vi "NML GPIB Tester.vi"(5 "String to write":string, 7 "Read":bool, 8 "Write":bool, 9 "VISA resource name":refnum<visa-resource-name>) -> (4 "String Read":string)   [LabVIEW 2024]
doc: "General LabView-GPIB VI which allows the selection of a message termination mode, timeout and usefule english error codes and status messages.\nScott Hannahs, FBNML, Feb 1993"
uses:
  <vilib>/Instr/_visa.llb/VISA GPIB Control REN Mode.ctl
panel:
  out "∆ Time (mS)":u32
  in  "Read Mode":u32(slide) scale=0.0..2.0
  in  "Write Mode":u32(slide) scale=0.0..5.0
  out "Error Out":errorcluster {"code" format="%.0x"}
  out "Write Status":string
  out "Read Status":string
  in  "Timeout (sec)":ext=1.0 format="%.1f"
  in  "Byte count":u32=2000
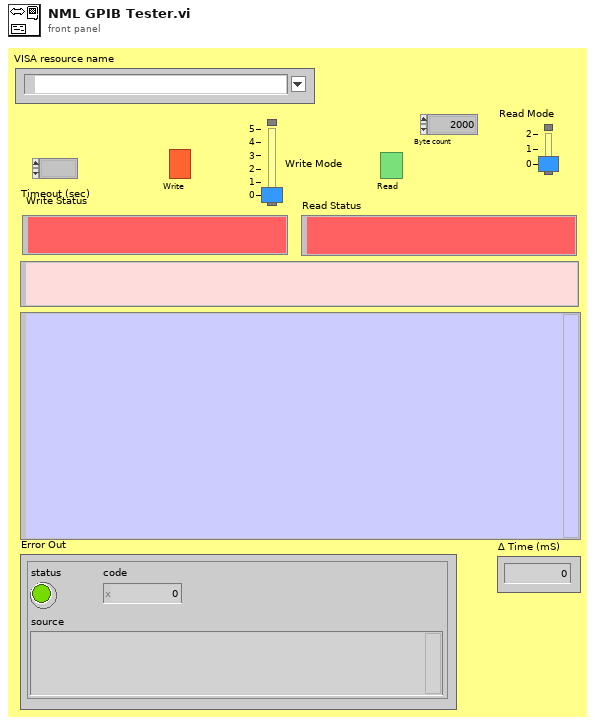
[diagram p1: front panel]
types:
  T1 = typedef "VISA GPIB Control REN Mode.ctl" = u16
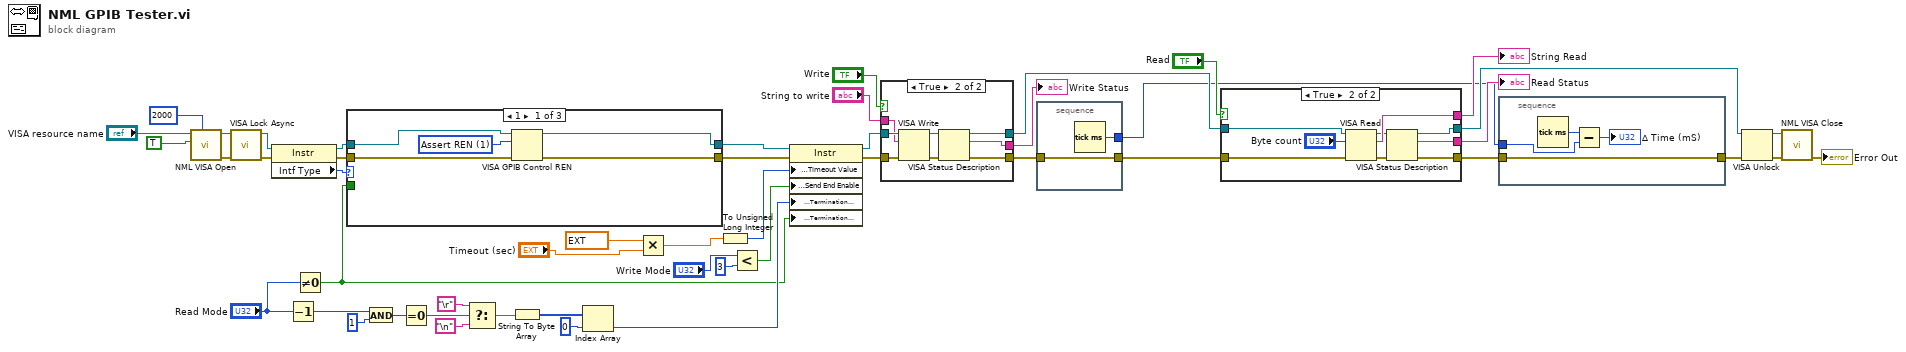
[diagram p0: block diagram]
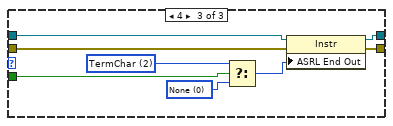
[diagram p3: hidden frame]
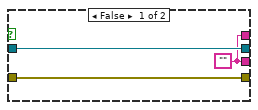
[diagram p4: hidden frame]
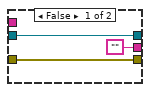
[diagram p5: hidden frame]
diagram:
  n1 = call "NML VISA Open.vi"("VISA Open timeout (0)"=u32 2000 ("timeout (0)"), "duplicate session (T)"=TRUE ("duplicate session (F)"), "VISA resource name"="VISA resource name") -> ("error out"=w8:errorcluster, "VISA resource name out"=w13:refnum<visa-resource-name>)  [unwired: 7 in]
  n2 = call <vilib>:"VISA Lock Async.vi"("error in (no error)"=w8, "VISA resource name"=w13) -> ("error out"=w7:errorcluster, "VISA resource name out"=w9:refnum<visa-resource-name>)  [unwired: 7 in, 1 out]
  n3 = property class="Instr"(reference=w9, error in=w7) -> (reference out=w11:refnum<visa-resource-name>, error out=w12:errorcluster, "Intf Type"=w2:u16)
  n4 = Decrement(x="Read Mode") -> (x-1=w29:u32)
  n5 = Not Equal To 0?(x="Read Mode") -> (x != 0?=w4:bool)
  n6 = case shown="1" w2 {
    tunnel: [w54 w56 w62] -> w15
    tunnel: [w53 w55 w61] -> w14
    tunnel: w12 -> [w52 w55 w63]
    tunnel: w11 -> [w51 w56 w64]
    tunnel: w4 -> [_ _ w58]
    frame 1 {
      w50 = T1 1 items=["Deassert REN", "Assert REN", "Go To Local; Deassert REN ", "Assert REN; Address Device", "Local Lockout (Addressed Devices)", "Local Lockout (This Device)", "Go To Local"] ("Mode")
      n7 = VISA GPIB Control REN(8:w52, 10:w50, 11:w51) -> (0:w53:errorcluster, 3:w54:refnum<visa-resource-name>)
    }
    frame Default {
    }
    frame 4 {
      w57 = u16 2 items=["None", "Last Bit", "TermChar", "Break"] ("Serial Settings:End Mode for Writes")
      w59 = u16 0 items=["None", "Last Bit", "TermChar", "Break"] ("Serial Settings:End Mode for Writes")
      n8 = Select(t=w57, s=w58, f=w59) -> (s? t:f=w60:u16)
      n9 = property class="Instr"(reference=w64, error in=w63, "ASRL End Out"=w60) -> (reference out=w62:refnum<visa-resource-name>, error out=w61:errorcluster)
    }
  }
  n10 = And(x=w29, y=u32 1) -> (x .and. y?=w31:u32)
  n11 = Equal To 0?(x=w31) -> (x = 0?=w32:bool)
  n12 = Select(t="\r", s=w32, f="\n") -> (s? t:f=w27:string)
  n13 = String To Byte Array(string=w27) -> (unsigned byte array=w26:u8[])
  n14 = Index Array(array=w26, index=0 ("Index")) -> (element=w22:u8)
  n15 = Multiply(x=ext 1000.0, y="Timeout (sec)") -> (x*y=w47:ext)
  n16 = To Unsigned Long Integer(number=w47) -> (unsigned 32bit integer=w41:u32)
  n17 = Less?(x="Write Mode", y=u32 3) -> (x < y?=w36:bool)
  n18 = property class="Instr"(reference=w15, error in=w14, "General Settings:Timeout Value"=w41, "Message Based Settings:Send End Enable"=w36, "Message Based Settings:Termination Character"=w22, "Message Based Settings:Termination Character Enable"=w4) -> (reference out=w39:refnum<visa-resource-name>, error out=w40:errorcluster)
  n19 = case shown="True" "Write" {
    tunnel: w39 -> [w67 w75]
    tunnel: w40 -> [w66 w74]
    tunnel: [w67 w72] -> w44
    tunnel: [w66 w70] -> w20
    tunnel: ["" w69] -> w24
    tunnel: "String to write" -> [_ w68]
    frame False {
    }
    frame True {
      n20 = VISA Write(VISA resource name=w75, write buffer=w68, error in (no error)=w74) -> (VISA resource name out=w73:refnum<visa-resource-name>, error out=w71:errorcluster)  [unwired: 1 out]
      n21 = VISA Status Description(8:w71, 11:w73) -> (0:w70:errorcluster, 2:w69:string, 3:w72:refnum<visa-resource-name>)
    }
  }
  "Write Status" <- w24
  n22 = stacked-sequence {
    tunnel: w20 -> [w77]
    tunnel: [w77] -> w19
    tunnel: [w76] -> w18
    frame #0 {
      n23 = Tick Count (ms)() -> (millisecond timer value=w76:u32)
    }
  }
  n24 = case shown="True" "Read" {
    tunnel: w44 -> [w79 w86]
    tunnel: w19 -> [w80 w87]
    tunnel: [w80 w84] -> w17
    tunnel: [w79 w83] -> w23
    tunnel: [w78 w89] -> w42
    tunnel: [w78 w81] -> w21
    frame False {
      w78 = ""
    }
    frame True {
      n25 = VISA Read(VISA resource name=w86, byte count="Byte count", error in (no error)=w87) -> (VISA resource name out=w82:refnum<visa-resource-name>, read buffer=w89:string, error out=w85:errorcluster)  [unwired: 1 out]
      n26 = VISA Status Description(8:w85, 11:w82) -> (0:w84:errorcluster, 2:w81:string, 3:w83:refnum<visa-resource-name>)
    }
  }
  "String Read" <- w42
  "Read Status" <- w21
  n27 = stacked-sequence {
    tunnel: w17 -> [w93]
    tunnel: [w93] -> w1
    tunnel: w18 -> [w90]
    frame #0 {
      n28 = Tick Count (ms)() -> (millisecond timer value=w92:u32)
      n29 = Subtract(x=w92, y=w90) -> (x-y=→"∆ Time (mS)":u32)
    }
  }
  n30 = VISA Unlock(8:w1, 11:w23) -> (0:w5:errorcluster, 3:w6:refnum<visa-resource-name>)
  n31 = call "NML VISA Close.vi"("Error In"=w5, "VISA resource name"=w6) -> ("Error Out"=→"Error Out":errorcluster)  [unwired: 9 in]
